vi "Append Incoming Bytes.vi"(7 "MQTT Version (3.1.1)":refnum<class "MQTTVersion.lvclass">, 8 "error in (no error)":errorcluster, 10 "Incoming Packets":u8[](array[numeric]) format="%08b", 11 "Incomplete ControlPacket":refnum<class "ControlPacket.lvclass">) -> (0 "error out":errorcluster, 1 "Complete Packet":bool, 2 "Remaining Packets":u8[](array[numeric]) format="%08b", 3 "ControlPacket":refnum<class "ControlPacket.lvclass">)   [LabVIEW 2013, in "MQTT_Control_Packets.lvlib" / "ControlPacket.lvclass"]
uses:
  ControlPacket.lvclass
  MQTT_311/MQTTVersion.lvclass
  ControlPacket.lvclass/ControlPacket.ctl
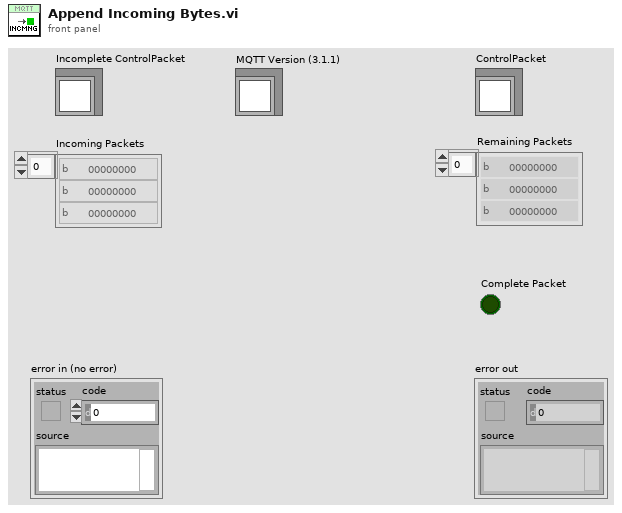
[diagram p1: front panel]
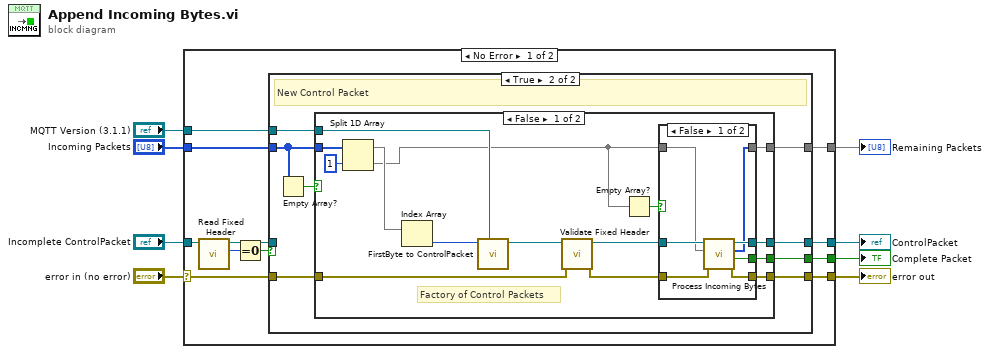
[diagram p0: block diagram]
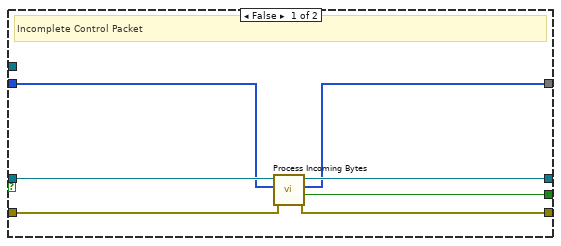
[diagram p2: hidden frame]
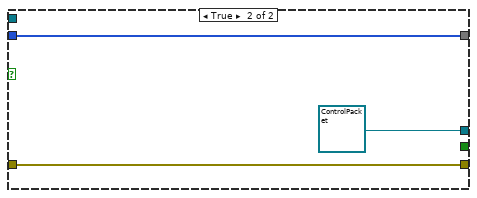
[diagram p4: hidden frame]
diagram:
  n1 = case shown="No Error" "error in (no error)" {
    selector: "error in (no error)" -> [w13 w65]
    tunnel: [w12 w65] -> w7
    tunnel: "Incomplete ControlPacket" -> [w19 w63]
    tunnel: "Incoming Packets" -> [w15 w64]
    tunnel: [w14 w63] -> w4
    tunnel: [w11 w64] -> w3
    tunnel: [w10 _] -> w2
    tunnel: "MQTT Version (3.1.1)" -> [w9 _]
    frame No Error {
      n2 = call "Read Fixed Header.vi"("ControlPacket in"=w19) -> ("Fixed Header"=w18:u8, "ControlPacket out"=w16:refnum<class "ControlPacket.lvclass">)  [unwired: 9 in]
      n3 = Equal To 0?(x=w18) -> (x = 0?=w17:bool)
      n4 = case shown="True" w17 {
        tunnel: w16 -> [w26 _]
        tunnel: w15 -> [w24 w29]
        tunnel: [w25 w33] -> w14
        tunnel: w13 -> [w22 w34]
        tunnel: [w21 w32] -> w12
        tunnel: [w23 w31] -> w11
        tunnel: [w20 w30] -> w10
        tunnel: w9 -> [_ w27]
        frame False {
          # "Incomplete Control Packet"
          n5 = call "Process Incoming Bytes.vi"("error in (no error)"=w22, "Incoming Packets"=w24, "ControlPacket in"=w26) -> ("error out"=w21:errorcluster, "Complete?"=w20:bool, "Remaining Packets"=w23:u8[], "ControlPacket out"=w25:refnum<class "ControlPacket.lvclass">)  [unwired: 5 in]
        }
        frame True {
          # "New Control Packet"
          n6 = Empty Array?(array=w29) -> (empty?=w28:bool)
          n7 = case shown="False" w28 {
            tunnel: w34 -> [w42 w61]
            tunnel: [w49 refnum<class "ControlPacket.lvclass"> refnum ("ControlPacket.lvclass")] -> w33
            tunnel: [w48 w61] -> w32
            tunnel: [w47 w62] -> w31
            tunnel: [w46 _] -> w30
            tunnel: w29 -> [w44 w62]
            tunnel: w27 -> [w37 _]
            frame False {
              # "Factory of Control Packets"
              n8 = Split 1D Array(array=w44, index=1 ("length")) -> (first subarray=w45:u8[], second subarray=w36:u8[])
              n9 = Index Array(array=w45) -> (element=w39:u8)  [unwired: 1 in]
              n10 = call-dynamic "FirstByte to ControlPacket.vi"("MQTTVersion"=w37, "Packet First Byte"=w39) -> ("Packet Type"=w38:refnum<class "ControlPacket.lvclass">)  [unwired: 9 in]
              n11 = call-dynamic "Validate Fixed Header.vi"("error in (no error)"=w42, "ControlPacket in"=w38) -> ("error out"=w41:errorcluster, "ControlPacket out"=w40:refnum<class "ControlPacket.lvclass">)  [unwired: 7 in, 1 out]
              n12 = Empty Array?(array=w36) -> (empty?=w35:bool)
              n13 = case shown="False" w35 {
                tunnel: [w56 w58] -> w49
                tunnel: [w55 w57] -> w48
                tunnel: [w54 w59] -> w47
                tunnel: [w53 _] -> w46
                tunnel: w41 -> [w52 w57]
                tunnel: w40 -> [w51 w58]
                tunnel: w36 -> [w50 w59]
                frame False {
                  n14 = call "Process Incoming Bytes.vi"("error in (no error)"=w52, "Incoming Packets"=w50, "ControlPacket in"=w51) -> ("error out"=w55:errorcluster, "Complete?"=w53:bool, "Remaining Packets"=w54:u8[], "ControlPacket out"=w56:refnum<class "ControlPacket.lvclass">)  [unwired: 5 in]
                }
                frame True {
                }
              }
            }
            frame True {
            }
          }
        }
      }
    }
    frame Error {
    }
  }
  "error out" <- w7
  "ControlPacket" <- w4
  "Complete Packet" <- w2
  "Remaining Packets" <- w3
